vi "Close Note File.vi"(8 "Error In":errorcluster, 10 "Notes":string, 11 "file path":path) -> (0 "Error Out":errorcluster)   [LabVIEW 2018]
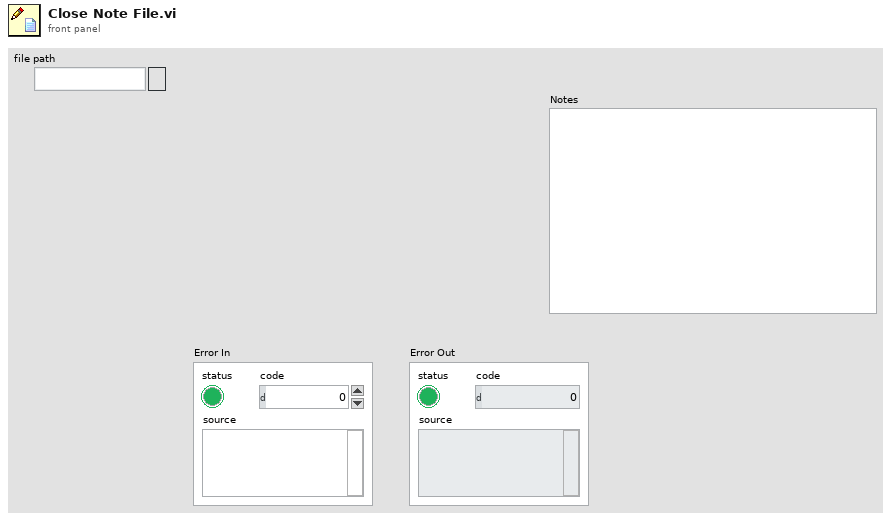
[diagram p1: front panel]
types:
  T1 = enum16{"open", "replace", "create", "open or create", "replace or create", "replace or create with confirmation"}
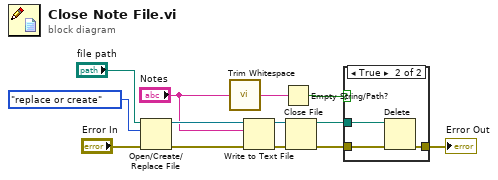
[diagram p0: block diagram]
diagram:
  n1 = Open/Create/Replace File(file path (use dialog)="file path", error in="Error In", operation (0:open)=T1."replace or create") -> (refnum out=w13:refnum<file>, error out=w12:errorcluster)  [unwired: 3 in, 1 out]
  n2 = call <vilib>:"Trim Whitespace.vi"("string"="Notes") -> ("trimmed string"=w2:string)  [unwired: 1 in]
  n3 = Write to Text File(file (use dialog)=w13, text="Notes", error in=w12) -> (refnum out=w11:refnum<file>, error out=w9:errorcluster)  [unwired: 1 in, 1 out]
  n4 = Empty String/Path?(string/path=w2) -> (empty?=w1:bool)
  n5 = Close File(refnum=w11, error in=w9) -> (path=w4:path, error out=w6:errorcluster)
  n6 = case shown="True" w1 {
    tunnel: w6 -> [w14 w17]
    tunnel: [w14 w16] -> w5
    tunnel: w4 -> [_ w15]
    frame False {
    }
    frame True {
      n7 = Delete(path (use dialog)=w15, error in=w17) -> (error out=w16:errorcluster)  [unwired: 3 in, 2 out]
    }
  }
  "Error Out" <- w5
